vi "Elevator Logic.vi"(8 "error in (no error)":errorcluster, 10 "Elevator Inputs":T1) -> (0 "error out":errorcluster, 2 "output":dbl format="%.2f")   [LabVIEW 2014]
uses:
  Elevator Input Data.ctl
  Elevator States.ctl
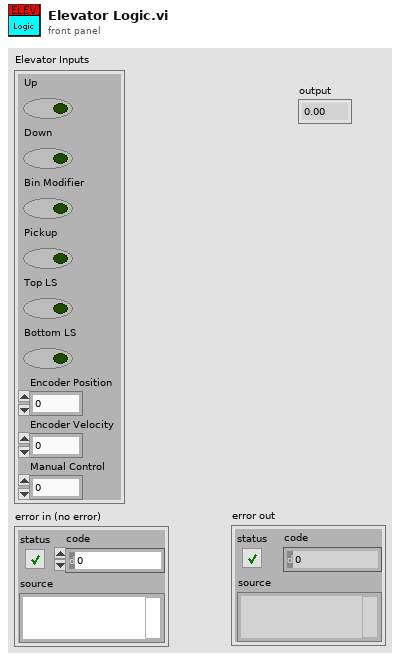
[diagram p1: front panel]
types:
  T1 = typedef "Elevator Input Data.ctl" = cluster{"Up":bool, "Down":bool, "Bin Modifier":bool, "Pickup":bool, "Top LS":bool, "Bottom LS":bool, "Encoder Position":dbl, "Encoder Velocity":dbl, "Manual Control":dbl}
  T2 = typedef "Elevator States.ctl" = enum16{"Ground", "Tote 1", "Tote 2", "Tote 3", "Tote 4", "Tote 5", "Tote 6"}
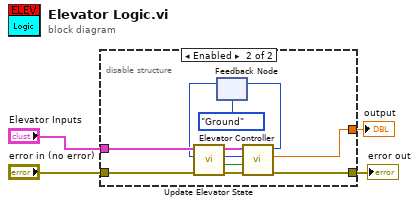
[diagram p0: block diagram]
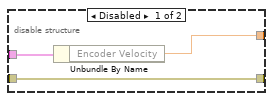
[diagram p2: hidden frame]
diagram:
  n1 = disable-structure shown="Enabled" {
    disable-tunnel: [w7 w11] -> w4
    disable-tunnel: "error in (no error)" -> [w7 w17]
    disable-tunnel: "Elevator Inputs" -> [w6 w16]
    disable-tunnel: [w5 w18] -> w1
    frame Disabled {
      n2 = Unbundle By Name(w6) -> ("Encoder Velocity"=w5:dbl)
    }
    frame Enabled {
      n3 = feedback #1(Elevator_States."Ground" ("State out")) -> (w9:T2)
      n4 = call "Update Elevator State.vi"("error in (no error)"=w17, "State in"=w9, "Elevator Inputs"=w16) -> ("error out"=w15:errorcluster, "Notify when settled?"=w12:bool, "State out"=w13:T2, "Elevator Inputs"=w14:T1)  [unwired: 5 in]
      n5 = call "Elevator Controller.vi"("error in (no error)"=w15, "Notify when settled?"=w12, "State in"=w13, "Elevator Inputs"=w14) -> ("error out"=w11:errorcluster, "Output"=w18:dbl, "State out"=w10:T2)  [unwired: 4 in, 1 out]
      n6 = feedback-in #1(w10) -> ()
    }
  }
  "error out" <- w4
  "output" <- w1
